vi "CSGToString.vi"(0 "Complex number":csg format="%#.20g", 5 "Precision":i16=6 caption="Precision (6)", 7 "Radix point":T1=enum."Comma (,)" caption="Radix point (,)", 9 "Remove trailing zeroes?":bool=TRUE caption="Remove trailing zeroes? (T)", 11 "Error in":errorcluster caption="Error in (no error)") -> (4 "String":string, 15 "Error out":errorcluster)   [LabVIEW 2017, in "GPString.lvlib"]
doc: "Converts <B>Complex number</B> to <B>String</B> observing the specified <B>Precision</B> and <B>Radix point</B>.\n\n<B>Radix point</B> can be either: System (localized), period (.), or comma (,).\n\nBy default this VI removes trailing zeroes in the fractional parts. Set <B>Remove trailing zeroes?</B> to False if you want to keep <B>Precision</B> number of digits in the fractional parts, even when the rightmost fractional digits are zeroes.\n\nThis VI is inlined and it runs only if there is no error on <B>Error in</B>.\n\nSteen Schmidt\nGPower\n15/6 2016"
uses:
  GPString.lvlib
  Typedefs/RadixPoint.ctl
panel:
  # "Copyright © 2016\nGPower\nSee enclosed license file for terms and conditions"
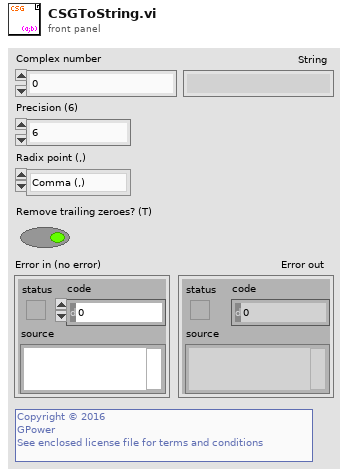
[diagram p1: front panel]
types:
  T1 = typedef "GPString.lvlib/RadixPoint.ctl" = enum16{"System", "Period (.)", "Comma (,)"}
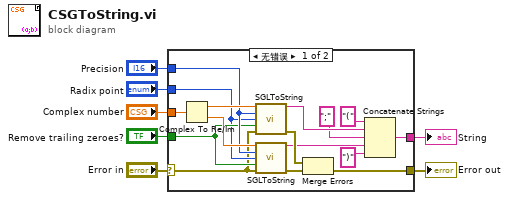
[diagram p0: block diagram]
diagram:
  n1 = case shown="无错误" "Error in" {
    selector: "Error in" -> [w10 w24]
    tunnel: "Complex number" -> [w23 _]
    tunnel: "Precision" -> [w20 _]
    tunnel: "Radix point" -> [w11 _]
    tunnel: [w9 w24] -> w4
    tunnel: [w13 _] -> w3
    tunnel: "Remove trailing zeroes?" -> [w12 _]
    frame No Error {
      n2 = Complex To Re/Im(x + iy=w23) -> (x=w22:sgl, y=w21:sgl)
      n3 = call "SGLToString.vi"("Number"=w22, "Precision"=w20, "Radix point"=w11, "Remove trailing zeroes?"=w12, "Error in"=w10) -> ("String"=w17:string, "Error out"=w19:errorcluster)  [unwired: 9 in]
      n4 = call "SGLToString.vi"("Number"=w21, "Precision"=w20, "Radix point"=w11, "Remove trailing zeroes?"=w12, "Error in"=w10) -> ("String"=w16:string, "Error out"=w18:errorcluster)  [unwired: 9 in]
      n5 = Merge Errors(w19, w18) -> (w9:errorcluster)
      n6 = Concatenate Strings("(", w17, ";" ("string"), w16, ")") -> (w13:string)
    }
    frame Error {
    }
  }
  "String" <- w3
  "Error out" <- w4
